vi "CH_LM App Select Meters.vi"(3 "Force selection?":bool) -> (0 "OK?":bool, 1 "Selected Meters":T1[](array[typedef]))   [LabVIEW 2012, in "CH_LM App.lvlib"]
doc: "This VI is a dialog to ask the user for a LabMax meter selection to used by the calling frontpanel instance."
uses:
  CH_LM App.lvlib
  CH_LM App Meter.ctl
  CH_LM.lvlib
panel:
  in  "Update":bool
  in  "Cancel":bool
  in  "OK":bool
  in  "Available Meters":i32[](listbox)
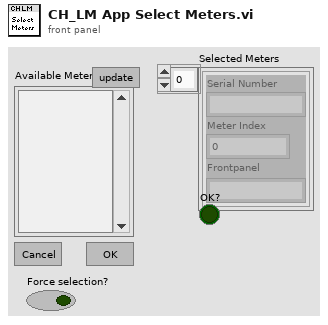
[diagram p1: front panel]
types:
  T1 = typedef "CH_LM App.lvlib/CH_LM App Meter.ctl" = cluster{"Serial Number":string, "Meter Index":i32, "Frontpanel":string}
  T2 = typedef "CH_LM.lvlib/CH_LM Meter Info.ctl" = cluster{"Meter Index":i32, "Serial Number":string, "Queue Cluster":T3, "Data Header":bool, "Data Tokens":T4[]}
  T3 = typedef "CH_LM.lvlib/CH_LM Queue Cluster.ctl" = cluster{"Streaming Queue":refnum<queue>, "Asynch Notifier":refnum<notifier>}
  T4 = typedef "CH_LM.lvlib/CH_LM Data Token.ctl" = enum16{"Raw data", "Quad distance", "Formated data", "Unit", "Pulse period", "Flags", "Sequence ID"}
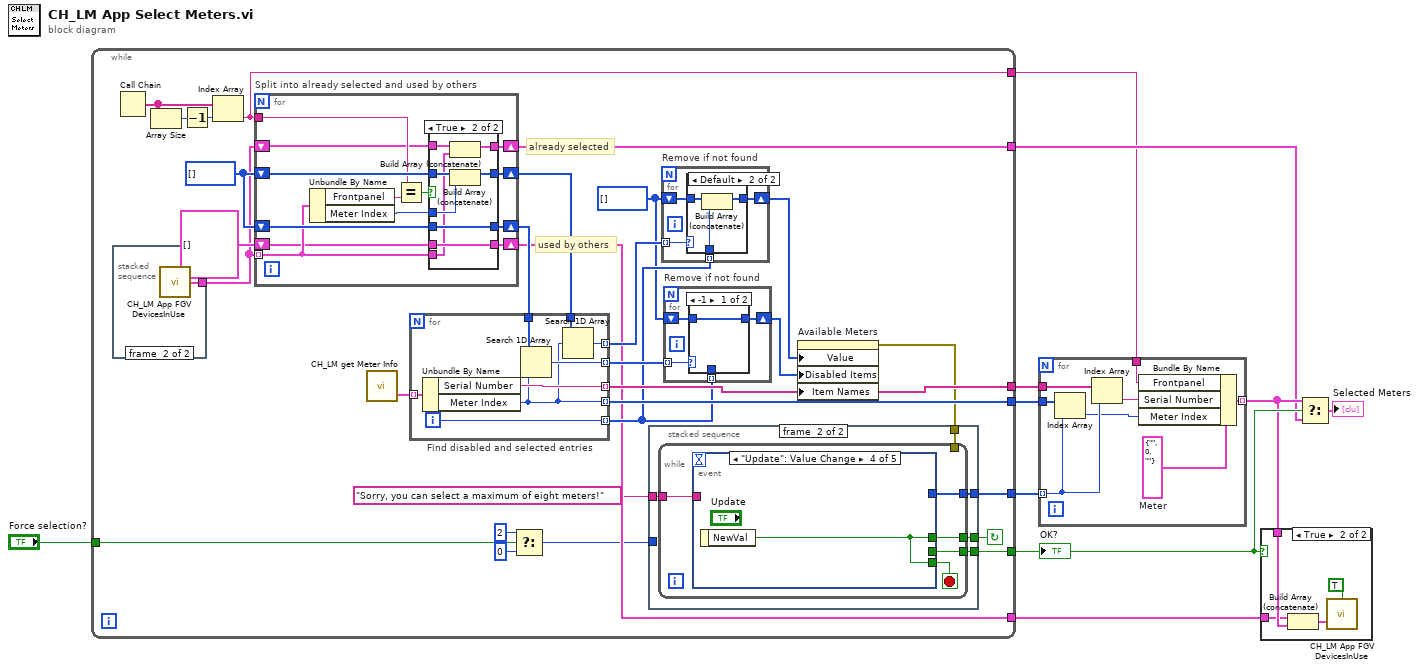
[diagram p0: block diagram]
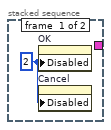
[diagram p2: hidden frame]
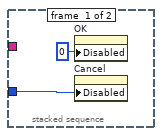
[diagram p3: hidden frame]
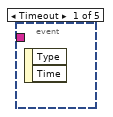
[diagram p4: hidden frame]
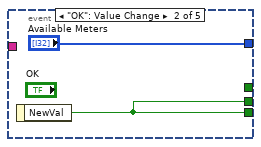
[diagram p5: hidden frame]
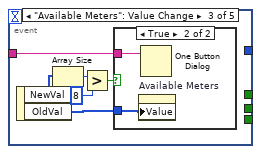
[diagram p6: hidden frame]
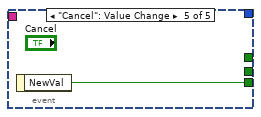
[diagram p8: hidden frame]
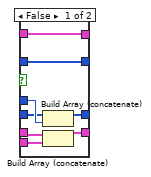
[diagram p10: hidden frame]
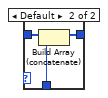
[diagram p11: hidden frame]
diagram:
  n1 = while {
    tunnel: [w38] -> w10
    tunnel: [w37] -> w9
    tunnel: [w34] -> w8
    tunnel: [w22] -> w7
    tunnel: [w19] -> w6
    tunnel: [w18] -> w3
    tunnel: [w17] -> w2
    tunnel: "Force selection?" -> [w13]
    stop <- w11 continue-if-true
    w30 = i32[] []
    w25 = i32[] []
    # "used by others"
    # "already selected"
    n2 = stacked-sequence {
      tunnel: [_ w41] -> w20
      frame #0 {
        w40 = u8 2 ("Disabled")
        n3 = property on="OK" class="Bool"("Disabled"=w40) -> ()  [unwired: 2 in, 2 out]
        n4 = property on="Cancel" class="Bool"("Disabled"=w40) -> ()  [unwired: 2 in, 2 out]
      }
      frame #1 {
        n5 = call "CH_LM App FGV DevicesInUse.vi"() -> ("Device Array"=w41:T1[])  [unwired: 2 in]
      }
    }
    n6 = Call Chain() -> (call chain=w33:string[])
    n7 = Array Size(array=w33) -> (size(s)=w32:i32)
    n8 = Decrement(x=w32) -> (x-1=w31:i32)
    n9 = Index Array(array=w33, index=w31) -> (element=w17:string)
    n10 = for "Split into already selected and used by others" {
      tunnel: w17 -> [w79]
      shift-right: [w82] -> w28
      shift-left: w30 -> [w83]
      shift-right: [w84] -> w29
      shift-left: w30 -> [w85]
      shift-right: [w77] -> w22
      shift-left: T1[] [] -> [w76]
      tunnel: w20 -> [w78] mode=indexing
      shift-right: [w75] -> w18
      shift-left: w20 -> [w74]
      n11 = Unbundle By Name(w78) -> ("Frontpanel"=w81:string, "Meter Index"=w80:i32)
      n12 = Equal?(x=w79, y=w81) -> (x = y?=w86:bool)
      n13 = case shown="True" w86 {
        tunnel: w85 -> [w91 w102]
        tunnel: w80 -> [w94 w101]
        tunnel: [w93 w102] -> w84
        tunnel: w83 -> [w92 w98]
        tunnel: [w92 w100] -> w82
        tunnel: w78 -> [w90 w97]
        tunnel: [w89 w99] -> w77
        tunnel: w76 -> [w88 w99]
        tunnel: [w87 w96] -> w75
        tunnel: w74 -> [w87 w95]
        frame False {
          n14 = Build Array (concatenate)(w91, w94) -> (w93:i32[])
          n15 = Build Array (concatenate)(w88, w90) -> (w89:T1[])
        }
        frame True {
          n16 = Build Array (concatenate)(w95, w97) -> (w96:T1[])
          n17 = Build Array (concatenate)(w98, w101) -> (w100:i32[])
        }
      }
    }
    n18 = call "CH_LM get Meter Info.vi"() -> ("All Meter Infos"=w39:T2[])  [unwired: 2 in, 9 out]
    n19 = for "Find disabled and selected entries" {
      tunnel: w39 -> [w118] mode=indexing
      tunnel: [w116] -> w38 mode=indexing
      tunnel: [w113] -> w34 mode=indexing
      tunnel: w29 -> [w117]
      tunnel: [w114] -> w36 mode=indexing
      tunnel: [w115] -> w26 mode=indexing
      tunnel: w28 -> [w112]
      tunnel: [w111] -> w27 mode=indexing
      i -> [w115]
      n20 = Unbundle By Name(w118) -> ("Serial Number"=w116:string, "Meter Index"=w113:i32)
      n21 = Search 1D Array(1D array=w117, element=w113) -> (index of element=w114:i32)  [unwired: 1 out]
      n22 = Search 1D Array(1D array=w112, element=w113) -> (index of element=w111:i32)  [unwired: 1 out]
    }
    n23 = Select(t=u8 2 ("Disabled"), s=w13, f=u8 0 ("Disabled")) -> (s? t:f=w12:u8)
    n24 = for "Remove if not found" {
      tunnel: w27 -> [w67] mode=indexing
      shift-right: [w69] -> w24
      shift-left: w25 -> [w68]
      tunnel: w26 -> [w66] mode=indexing
      n25 = case shown="Default" w67 {
        tunnel: [w70 w73] -> w69
        tunnel: w68 -> [w70 w72]
        tunnel: w66 -> [_ w71]
        frame -1 {
        }
        frame Default {
          n26 = Build Array (concatenate)(w72, w71) -> (w73:i32[])
        }
      }
    }
    n27 = for "Remove if not found" {
      tunnel: w36 -> [w104] mode=indexing
      shift-right: [w106] -> w35
      shift-left: w25 -> [w105]
      tunnel: w26 -> [w103] mode=indexing
      n28 = case shown="-1" w104 {
        tunnel: [w107 w110] -> w106
        tunnel: w105 -> [w107 w109]
        tunnel: w103 -> [_ w108]
        frame -1 {
        }
        frame Default {
          n29 = Build Array (concatenate)(w109, w108) -> (w110:i32[])
        }
      }
    }
    n30 = property on="Available Meters" class="LstBox (strict)"("Value"=w24, "Disabled Items"=w35, "Item Names"=w38) -> (error out=w23:errorcluster)  [unwired: 2 in, 1 out]
    n31 = stacked-sequence {
      tunnel: [_ w48] -> w37
      tunnel: [_ w47] -> w19
      tunnel: w23 -> [_ w46]
      tunnel: "Sorry, you can select a maximum of eight meters!" -> [_ w45]
      tunnel: w12 -> [w42 _]
      tunnel: [_ w44] -> w11
      frame #0 {
        n32 = property on="OK" class="Bool"("Disabled"=u8 0) -> ()  [unwired: 2 in, 2 out]
        n33 = property on="Cancel" class="Bool"("Disabled"=w42) -> ()  [unwired: 2 in, 2 out]
      }
      frame #1 {
        n34 = while {
          tunnel: [w52] -> w47
          tunnel: [w51] -> w48
          tunnel: w46 -> [_]
          tunnel: w45 -> [w50]
          tunnel: [w49] -> w44
          stop <- w53 stop-if-true
          n35 = event shown="[3] \"Update\": Value Change" {
            selector: _ -> [_ _ _ _ _]
            dyn-events: _ -> [_ _ _ _ _]
            timeout: _ -> [_ _ _ _ _]
            tunnel: [_ w55 _ w64 w65] -> w53
            tunnel: [_ w55 _ _ _] -> w52
            tunnel: [_ "Available Meters" _ _ _] -> w51
            tunnel: w50 -> [_ _ w56 _ _]
            tunnel: [_ _ _ w64 _] -> w49
            event Timeout {
              n36 = event-data() -> ()  [unwired: 3 out]
            }
            event "OK": Value Change {
              n37 = event-data() -> ("NewVal"=w55:bool)  [unwired: 1 out]
            }
            event "Available Meters": Value Change {
              n38 = event-data() -> ("NewVal"=w59:i32[], "OldVal"=w58:i32[])  [unwired: 1 out]
              n39 = Array Size(array=w59) -> (size(s)=w61:i32)
              n40 = Greater?(x=w61, y=8) -> (0:w57:bool)
              n41 = case shown="True" w57 {
                tunnel: w58 -> [_ w63]
                tunnel: w56 -> [_ w62]
                frame False {
                }
                frame True {
                  n42 = property on="Available Meters" class="LstBox (strict)"("Value"=w63) -> ()  [unwired: 2 in, 2 out]
                  n43 = One Button Dialog(message=w62) -> ()  [unwired: 2 out]
                }
              }
            }
            event "Update": Value Change {
              n44 = event-data() -> ("NewVal"=w64:bool)  [unwired: 1 out]
            }
            event "Cancel": Value Change {
              n45 = event-data() -> ("NewVal"=w65:bool)  [unwired: 1 out]
            }
          }
        }
      }
    }
  }
  "OK?" <- w6
  n46 = for {
    tunnel: w10 -> [w125]
    tunnel: w8 -> [w126]
    tunnel: w9 -> [w124] mode=indexing
    tunnel: [w123] -> w5 mode=indexing
    tunnel: w2 -> [w119]
    w122 = T1 {"Serial Number"="", "Meter Index"=0, "Frontpanel"=""}  # Meter
    n47 = Index Array(array=w126, index=w124) -> (element=w120:i32)
    n48 = Index Array(array=w125, index=w124) -> (element=w121:string)
    n49 = Bundle By Name(cluster=w122, "Frontpanel"=w119, "Serial Number"=w121, "Meter Index"=w120) -> (w123:T1)
  }
  n50 = case shown="True" w6 {
    tunnel: w5 -> [_ w128]
    tunnel: w7 -> [_ w127]
    frame False {
    }
    frame True {
      n51 = Build Array (concatenate)(w127, w128) -> (w130:T1[])
      n52 = call "CH_LM App FGV DevicesInUse.vi"("Device Array"=w130, "set? (F)"=TRUE) -> ()  [unwired: 1 out]
    }
  }
  n53 = Select(t=w5, s=w6, f=w3) -> (s? t:f=→"Selected Meters":T1[])
